vi "FTW-TestExecutive-Core_Initialize.vi"(0 "Test Executive":refnum<class "FTW-TestExecutive-Core.lvclass">, 5 "Initialization Sequence":string, 7 "FTW Actor Instance Configuration":string, 11 "error in (no error)":errorcluster) -> (4 "FTW-TestExecutive-Core Out":refnum<class "FTW-TestExecutive-Core.lvclass">, 6 "Event Refnums":T1, 10 "Refresh Period":dbl, 15 "error out":errorcluster)   [LabVIEW 2015, in "FTW-TestExecutive-Core.lvclass"]
uses:
  FTW-TestExecutive-Core.lvclass
  source/actor/Message/Request/FTW-Message-IncomingRequest.lvclass
  source/actor/Message/Base/FTW-Message.lvclass
  FTW-TestExecutive-Core.lvclass/FTW-TestExecutive-Core.ctl
  source/JSON/core/FTW-JSON-Core-EncodingFlags.vi
  source/JSON/FTW-JSON-Parse.vi
  source/Reflection/FTW-Reflection-Type.vi
  source/CodeGen/JSON Deserialize/FTW-JSON-Core-GetFlattenedValue.vi
  source/CodeGen/JSON Deserialize/FTW-JSON-Deserialize.xnode
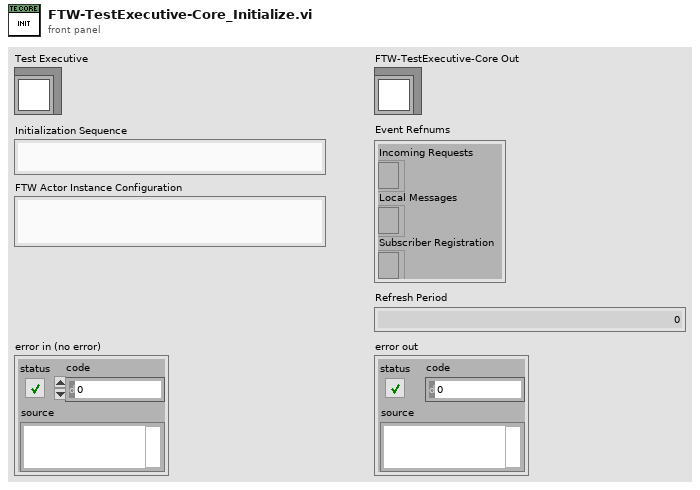
[diagram p1: front panel]
types:
  T1 = cluster{"Incoming Requests":refnum<event-registration>, "Local Messages":refnum<event-registration>, "Subscriber Registration":refnum<event-registration>}
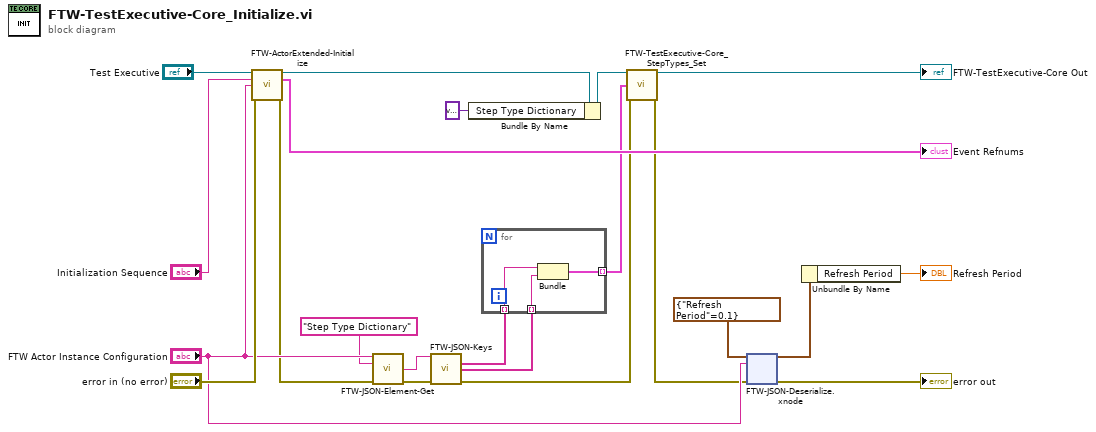
[diagram p0: block diagram]
diagram:
  n1 = call-dynamic "FTW-ActorExtended-Initialize.vi"("FTW Actor Instance Type"="Test Executive", "Initialization Job Sequence"="Initialization Sequence", "Actor Instance Configuration"="FTW Actor Instance Configuration", "error in"="error in (no error)") -> ("FTW Actor Instance"=w6:refnum<class "FTW-TestExecutive-Core.lvclass">, "Event Refnums"=→"Event Refnums":T1, "error out"=w10:errorcluster)  [unwired: 9 in]
  n2 = call "FTW-JSON-Element-Get.vi"("JSON Opject"="FTW Actor Instance Configuration", "Key"="Step Type Dictionary", "error in"=w10) -> ("Element"=w12:string, "error out"=w11:errorcluster)  [unwired: 10 in, 1 out]
  n3 = call "FTW-JSON-Keys.vi"("JSON Opject"=w12, "error in"=w11) -> ("Keys"=w9:string[], "Values"=w8:string[], "error out"=w2:errorcluster)  [unwired: 11 in]
  n4 = Bundle By Name(cluster=w6, "Step Type Dictionary"=variant) -> (w4:refnum<class "FTW-TestExecutive-Core.lvclass">)
  n5 = for {
    tunnel: w9 -> [w25] mode=indexing
    tunnel: w8 -> [w24] mode=indexing
    tunnel: [w23] -> w7 mode=indexing
    n6 = Bundle("String"=w25, "String"=w24) -> (w23:cluster{"String":string, "String":string})  [unwired: 1 in]
  }
  n7 = call "FTW-TestExecutive-Core_StepTypes_Set.vi"("FTW-TestExecutive-Core In"=w4, "Step Types"=w7, "error in"=w2) -> ("FTW-TestExecutive-Core Out"=→"FTW-TestExecutive-Core Out":refnum<class "FTW-TestExecutive-Core.lvclass">, "error out"=w1:errorcluster)  [unwired: 11 in]
  n8 = xnode "FTW-JSON-Deserialize.xnode"("Type and Defaults"=cluster{"Refresh Period":dbl} {"Refresh Period"=0.1}, "JSON String"="FTW Actor Instance Configuration", "error in"=w1) -> ("Values"=w20:cluster{"Refresh Period":dbl}, "error out"=→"error out":errorcluster)
  n9 = Unbundle By Name(w20) -> ("Refresh Period"=→"Refresh Period":dbl)
